vi "Read AbsTimeOffset.vi"(8 "error in (no error)":errorcluster, 11 "NIScope in":refnum<class "NIScope.lvclass">) -> (0 "error out":errorcluster, 2 "AbsTimeOffset":dbl[](array[numeric]), 3 "NIScope out":refnum<class "NIScope.lvclass">)   [LabVIEW 2014, in "ScopePlugins.lvlib" / "NIScope.lvclass"]
uses:
  NIScope.lvclass
  NIScope.lvclass/NIScope.ctl
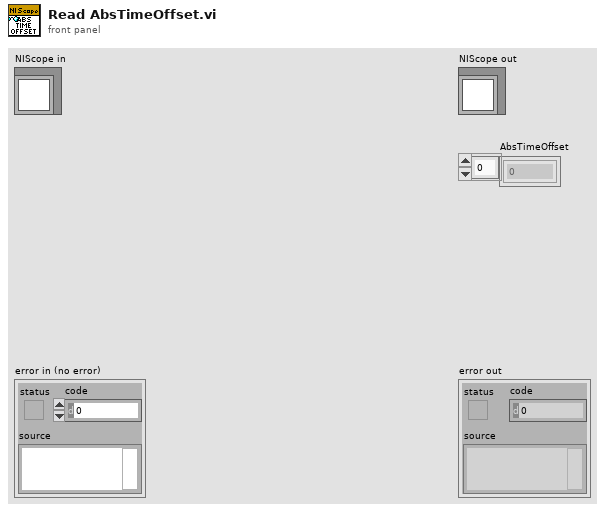
[diagram p1: front panel]
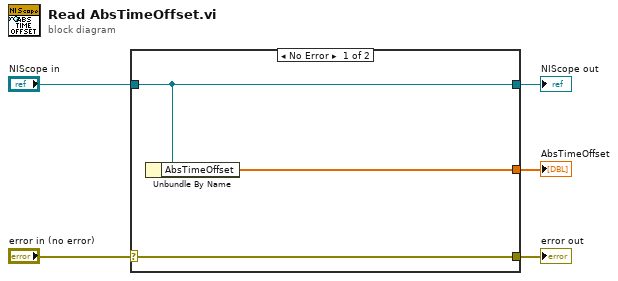
[diagram p0: block diagram]
diagram:
  n1 = case shown="No Error" "error in (no error)" {
    selector: "error in (no error)" -> [w8 w9]
    tunnel: [w8 w9] -> w4
    tunnel: [w7 w10] -> w2
    tunnel: "NIScope in" -> [w7 w10]
    tunnel: [w6 _] -> w1
    frame No Error {
      n2 = Unbundle By Name(w7) -> ("AbsTimeOffset"=w6:dbl[])
    }
    frame Error {
    }
  }
  "error out" <- w4
  "NIScope out" <- w2
  "AbsTimeOffset" <- w1
